vi "componentSimulator.vi"(8 "error in":errorcluster) -> (0 "error out":errorcluster)   [LabVIEW 2018]
doc: "Simulate a software component that will use the Tcp Server."
uses:
  src/TcpServer/TcpServer.lvclass
  src/TcpServer/TcpServer.lvclass/TcpServer.ctl
  src/TcpServer/eventTypeDef.ctl
  src/TcpServer/runServer.vi
panel:
  out "json_cmd":string
  in  "Tab Control":T1(tab)
  out "confData":T2={"clientIP"="127.0.0.1", "serverPort"=8888, "serverTimeout (ms)"=100, "serverBytesToRead"=32768} caption="Server Configurations"
  in  "fail":bool
  in  "success":bool
  in  "send_event":bool
  in  "evtName":string="event3" caption="Event Name"
  in  "stop_server":bool
  in  "Stop Simulator":bool caption="stop"
  # "Component Simulator"
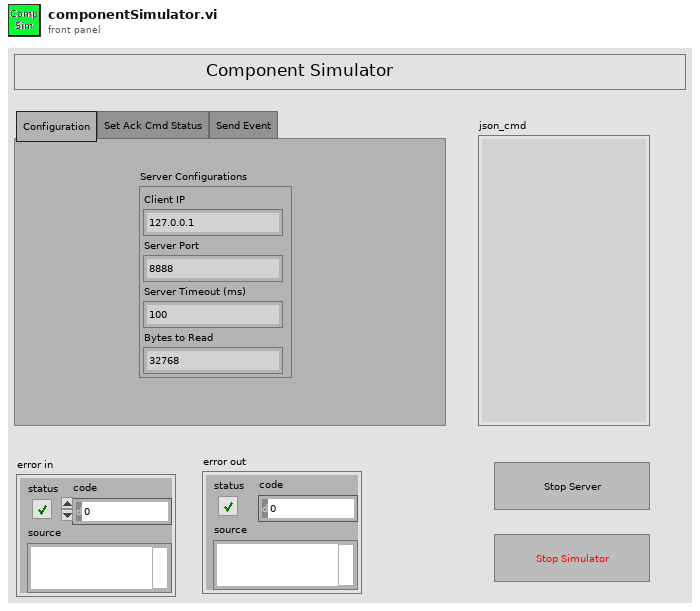
[diagram p1: front panel]
types:
  T1 = enum32{"Configuration", "Set Ack Cmd Status", "Send Event"}
  T2 = cluster{"clientIP":string, "serverPort":u16, "serverTimeout (ms)":i32, "serverBytesToRead":i32}
  T3 = typedef "userEventsTypeDef.ctl" = cluster{"TcpServer":refnum<user-event>, "Command":refnum<user-event>, "CmdStatus":refnum<user-event>, "Event":refnum<user-event>, "Telemetry":refnum<user-event>}
  T4 = typedef "TcpServer.lvclass/eventTypeDef.ctl" = cluster{"evtName":string, "evt_details":cluster{"state":i32}}
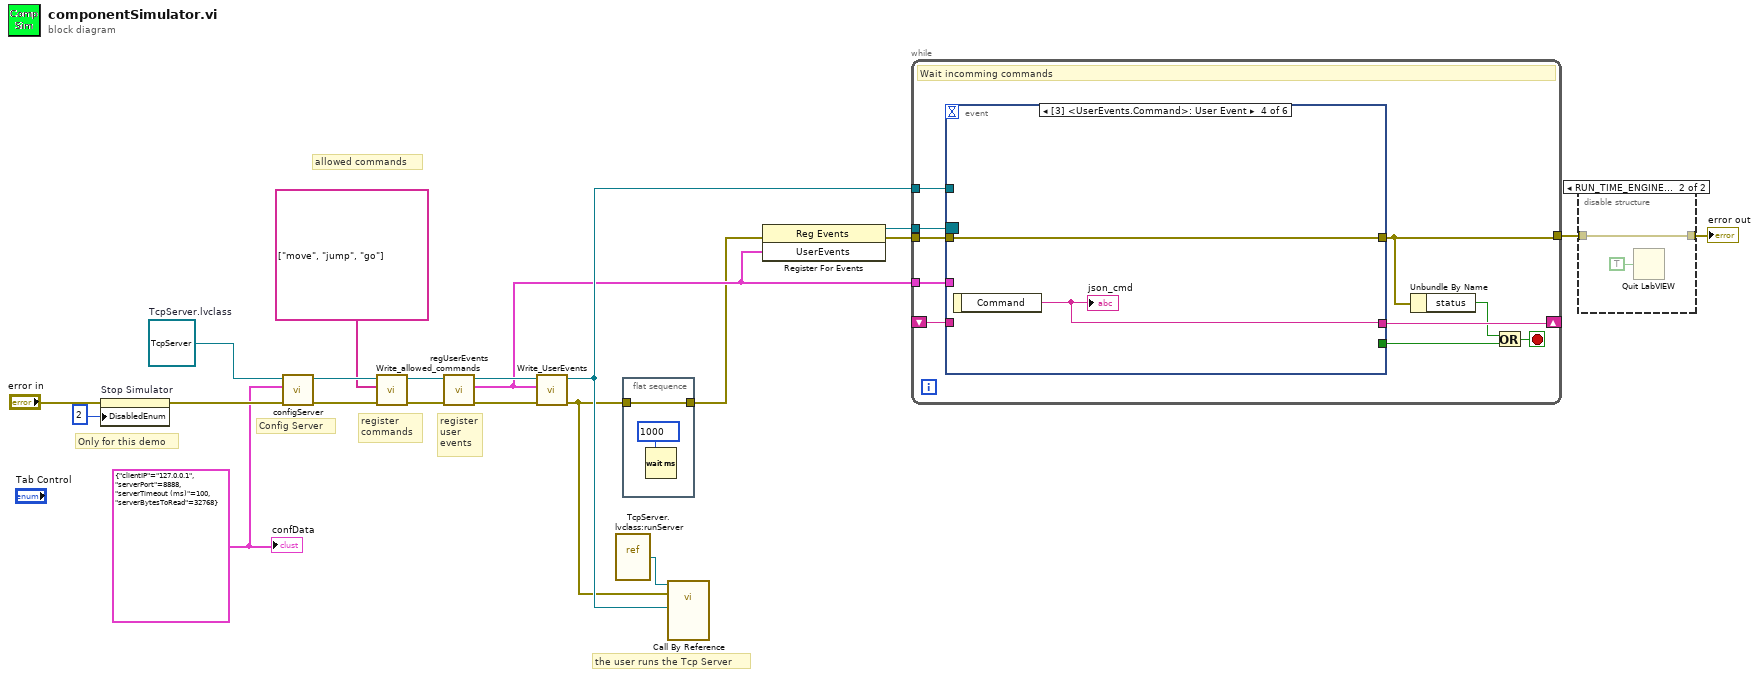
[diagram p0: block diagram]
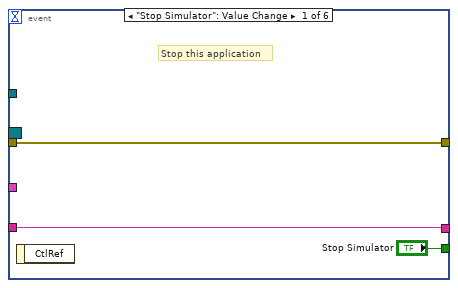
[diagram p3: hidden frame]
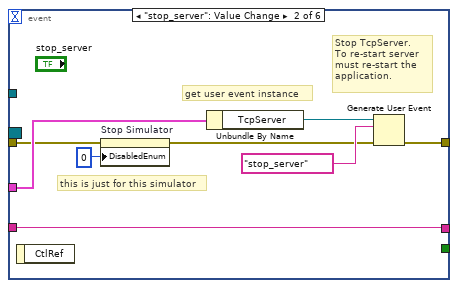
[diagram p4: hidden frame]
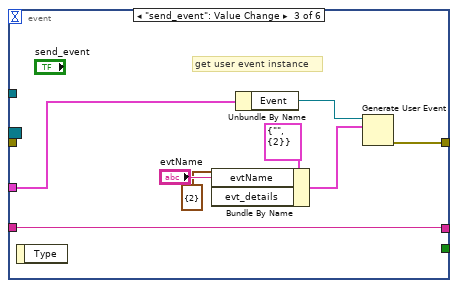
[diagram p5: hidden frame]
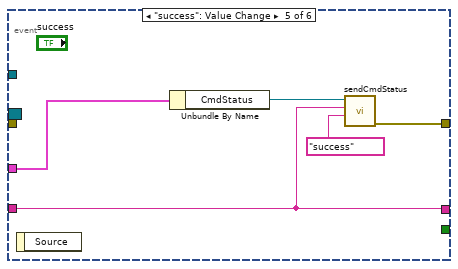
[diagram p6: hidden frame]
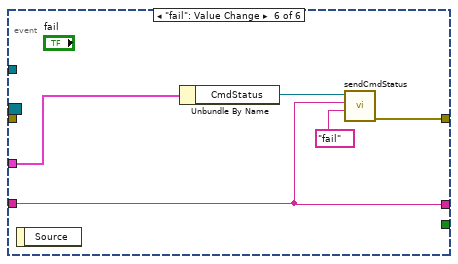
[diagram p7: hidden frame]
diagram:
  w13 = T2 {"clientIP"="127.0.0.1", "serverPort"=8888, "serverTimeout (ms)"=100, "serverBytesToRead"=32768} ("confData")
  w14 = refnum<class "TcpServer.lvclass"> refnum  # TcpServer.lvclass
  # "register\nuser\nevents"
  # "register \ncommands"
  # "allowed commands"
  # "the user runs the Tcp Server"
  # "Config Server"
  # "Only for this demo"
  n1 = property on="Stop Simulator" class="Bool"(error in="error in", "DisabledEnum"=2) -> (error out=w15:errorcluster)  [unwired: 1 in, 1 out]
  n2 = call "configServer.vi"("error in (no error)"=w15, "confData"=w13, "tcpServer in"=w14) -> ("error out"=w12:errorcluster, "tcpServer out"=w5:refnum<class "TcpServer.lvclass">)  [unwired: 7 in]
  n3 = call "Write_allowed_commands.vi"("error in (no error)"=w12, "allowed_commands"=string[] ["move", "jump", "go"], "TcpServer in"=w5) -> ("error out"=w6:errorcluster, "TcpServer out"=w4:refnum<class "TcpServer.lvclass">)  [unwired: 7 in]
  n4 = call "regUserEvents.vi"("error in (no error)"=w6, "tcpServer in"=w4) -> ("error out"=w9:errorcluster, "UserEvents"=w7:T3, "tcpServer out"=w8:refnum<class "TcpServer.lvclass">)  [unwired: 7 in]
  n5 = call "Write_UserEvents.vi"("error in (no error)"=w9, "UserEvents"=w7, "TcpServer in"=w8) -> ("error out"=w2:errorcluster, "TcpServer out"=w11:refnum<class "TcpServer.lvclass">)  [unwired: 7 in]
  n6 = vi-ref "TcpServer.lvclass:runServer.vi"() -> (w10:refnum<vi>)
  n7 = flat-sequence {
    tunnel: w2 -> [w22]
    tunnel: [w22] -> w1
    frame #0 {
      n8 = Wait (ms)(milliseconds to wait=u32 1000) -> ()  [unwired: 1 out]
    }
  }
  n9 = call-by-ref "?"(reference=w10, error in=w2, "TcpServer in"=w11) -> ()  [unwired: 9 in, 4 out]
  n10 = register-events(error in=w1, w7) -> (reference out=w17:refnum<event-registration>, error out=w16:errorcluster)  [unwired: 1 in]
  n11 = while {
    tunnel: w16 -> [w33]
    tunnel: [w25] -> w21
    tunnel: w17 -> [w32]
    tunnel: w11 -> [w31]
    tunnel: w7 -> [w30]
    shift-right: [w29] -> _
    shift-left: _ -> [w28]
    stop <- w27 stop-if-true
    # "Wait incomming commands"
    n12 = event shown="[3] <UserEvents.Command>: User Event" {
      selector: w32 -> [_ _ _ _ _ _]
      dyn-events: _ -> [_ _ _ _ _ _]
      timeout: _ -> [_ _ _ _ _ _]
      tunnel: ["Stop Simulator" _ _ _ _ _] -> w26
      tunnel: [w35 w42 w48 w53 w55 w60] -> w25
      tunnel: w33 -> [w35 w38 _ w53 _ _]
      tunnel: w31 -> [_ _ _ _ _ _]
      tunnel: w30 -> [_ w40 w45 _ w59 w64]
      tunnel: [w34 w41 w46 w54 w56 w61] -> w29
      tunnel: w28 -> [w34 w41 w46 _ w56 w61]
      event "Stop Simulator": Value Change {
        # "Stop this application"
        n13 = event-data() -> ()  [unwired: 1 in, 1 out]
      }
      event "stop_server": Value Change {
        # "Stop TcpServer.\nTo re-start server \nmust re-start the \napplication."
        # "this is just for this simulator"
        # "get user event instance"
        n14 = event-data() -> ()  [unwired: 1 in, 1 out]
        n15 = property on="Stop Simulator" class="Bool"(error in=w38, "DisabledEnum"=0) -> (error out=w37:errorcluster)  [unwired: 1 in, 1 out]
        n16 = Unbundle By Name(w40) -> ("TcpServer"=w39:refnum<user-event>)
        n17 = Generate User Event(user event=w39, event data cluster="stop_server" ("event data"), error in=w37) -> (error out=w42:errorcluster)  [unwired: 1 in, 1 out]
      }
      event "send_event": Value Change {
        # "get user event instance"
        n18 = event-data() -> ()  [unwired: 1 in, 1 out]
        n19 = Bundle By Name(cluster=T4 {"evtName"="", "evt_details"={"state"=2}}, "evtName"="evtName", "evt_details"=cluster{"state":i32} {"state"=2}) -> (w49:T4)
        n20 = Unbundle By Name(w45) -> ("Event"=w52:refnum<user-event>)
        n21 = Generate User Event(user event=w52, event data cluster=w49) -> (error out=w48:errorcluster)  [unwired: 2 in, 1 out]
      }
      event User Event {
        n22 = event-data() -> ("Command"=w54:string)  [unwired: 1 in]
        "json_cmd" <- w54
      }
      event "success": Value Change {
        n23 = event-data() -> ()  [unwired: 1 in, 1 out]
        n24 = Unbundle By Name(w59) -> ("CmdStatus"=w57:refnum<user-event>)
        n25 = call "sendCmdStatus.vi"("cmdStatus"="success", "json_command"=w56, "user event"=w57) -> ("error out"=w55:errorcluster)  [unwired: 8 in]
      }
      event "fail": Value Change {
        n26 = event-data() -> ()  [unwired: 1 in, 1 out]
        n27 = Unbundle By Name(w64) -> ("CmdStatus"=w62:refnum<user-event>)
        n28 = call "sendCmdStatus.vi"("cmdStatus"="fail", "json_command"=w61, "user event"=w62) -> ("error out"=w60:errorcluster)  [unwired: 8 in]
      }
    }
    n29 = Unbundle By Name(w25) -> ("status"=w24:bool)
    n30 = Or(x=w24, y=w26) -> (x .or. y?=w27:bool)
  }
  n31 = disable-structure shown="RUN_TIME_ENGINE==True" {
    disable-tunnel: w21 -> [w65 w66]
    disable-tunnel: [w65 w66] -> w20
    frame condition #0 (active) {
    }
    frame condition #1 {
      n32 = Quit LabVIEW(quit? (T)=TRUE) -> ()
    }
  }
  "error out" <- w20
  "confData" <- w13
